vi "Excel___Write Channel Grouping.vi"(0 "Sheets Ref In":refnum<k7>, 5 "Starting Row":i32, 7 "Data 1":string[][](array[string]), 9 "Data 2":string[][](array[string]), 11 "Error In":errorcluster) -> (4 "Sheets Ref Out":refnum<k7>, 15 "Error Out":errorcluster)   [LabVIEW 2013]
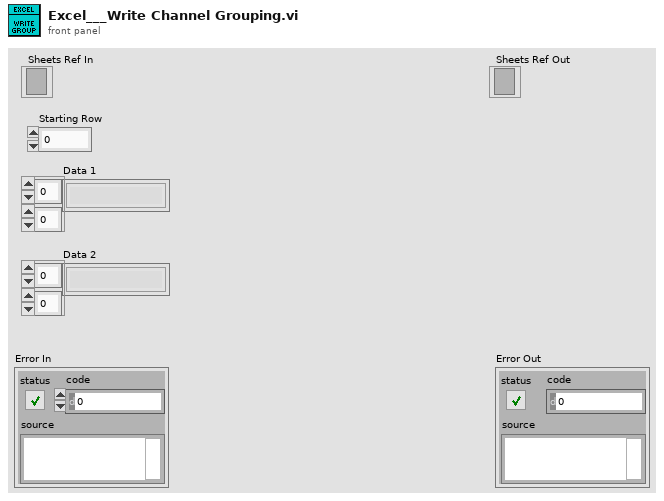
[diagram p1: front panel]
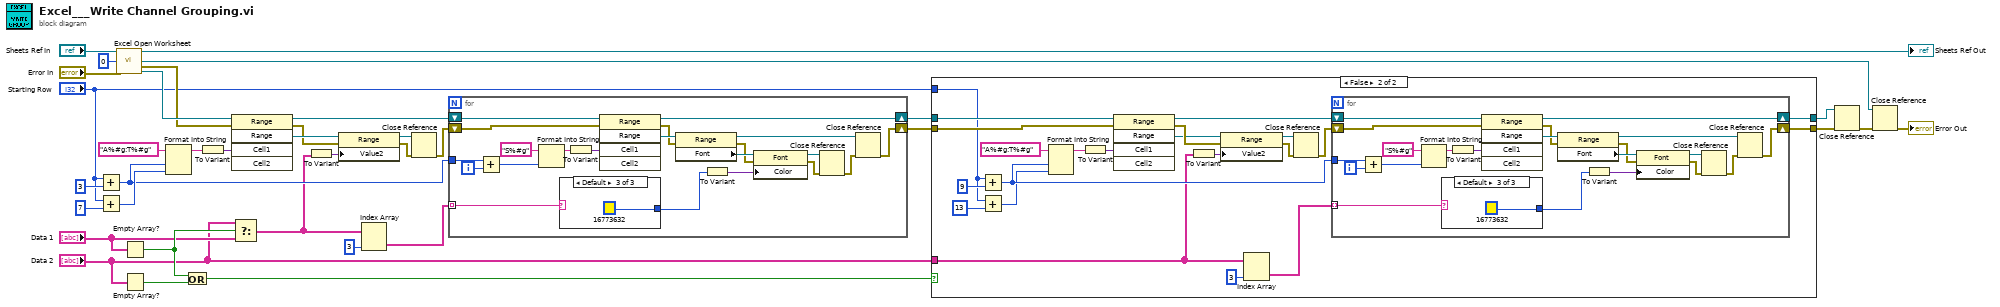
[diagram p0: block diagram]
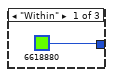
[diagram p3: hidden frame]
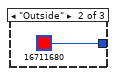
[diagram p4: hidden frame]
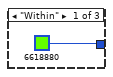
[diagram p5: hidden frame]
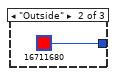
[diagram p6: hidden frame]
diagram:
  n1 = Add(x="Starting Row", y=3) -> (x+y=w13:i32)
  n2 = Add(x="Starting Row", y=7) -> (x+y=w19:i32)
  n3 = call "Excel Open Worksheet.vi"("Sheets Ref In"="Sheets Ref In", "Sheet#"=0, "Error In"="Error In") -> ("Sheets Ref Out"=→"Sheets Ref Out":refnum<k7>, "Worksheet Ref Out"=w27:refnum<k7>, "Error Out"=w23:errorcluster, "Cells Ref Out"=w24:refnum<k7>)  [unwired: 9 in]
  n4 = Empty Array?(array="Data 1") -> (empty?=w4:bool)
  n5 = Empty Array?(array="Data 2") -> (empty?=w6:bool)
  n6 = Format Into String(initial string="A%#g:T%#g", w13, w19) -> (resulting string=w35:string)  [unwired: 2 in, 1 out]
  n7 = Or(x=w4, y=w6) -> (x .or. y?=w5:bool)
  n8 = To Variant(anything=w35) -> (Variant=w34:variant)
  n9 = invoke class="Range" method="Range"(reference=w24, error in=w23, "Cell1"=w34) -> (reference out=w16:refnum<k7>, error out=w31:errorcluster, "Range"=w33:refnum<k7>)  [unwired: 2 in, 2 out]
  n10 = Select(t="Data 2", s=w4, f="Data 1") -> (s? t:f=w1:string[][])
  n11 = To Variant(anything=w1) -> (Variant=w32:variant)
  n12 = property class="Range"(reference=w33, error in=w31, "Value2"=w32) -> (reference out=w22:refnum<k7>, error out=w17:errorcluster)
  n13 = Index Array(array=w1, index (col)=3 ("disabled index (col)")) -> (element=w14:string[])  [unwired: 1 in]
  n14 = Close Reference(reference=w22, error in (no error)=w17) -> (error out=w15:errorcluster)
  n15 = for {
    tunnel: w14 -> [w46] mode=indexing
    shift-right: [w49] -> w12
    shift-left: w16 -> [w57]
    shift-right: [w37] -> w11
    shift-left: w15 -> [w56]
    tunnel: w13 -> [w53]
    i -> [w52]
    n16 = Add(x=w53, y=w52) -> (x+y=w51:i32)
    n17 = Format Into String(initial string="S%#g", w51) -> (resulting string=w55:string)  [unwired: 2 in, 1 out]
    n18 = case shown="Default" w46 {
      tunnel: [u32 6618880 u32 16711680 u32 16773632] -> w44
      frame "Within" {
      }
      frame "Outside" {
      }
      frame Default {
      }
    }
    n19 = To Variant(anything=w55) -> (Variant=w50:variant)
    n20 = invoke class="Range" method="Range"(reference=w57, error in=w56, "Cell1"=w50) -> (reference out=w49:refnum<k7>, error out=w43:errorcluster, "Range"=w48:refnum<k7>)  [unwired: 2 in, 2 out]
    n21 = property class="Range"(reference=w48, error in=w43) -> (reference out=w39:refnum<k7>, error out=w42:errorcluster, "Font"=w47:refnum<k7>)
    n22 = To Variant(anything=w44) -> (Variant=w45:variant)
    n23 = property class="Font"(reference=w47, error in=w42, "Color"=w45) -> (reference out=w40:refnum<k7>, error out=w41:errorcluster)
    n24 = Close Reference(reference=w40, error in (no error)=w41) -> (error out=w38:errorcluster)
    n25 = Close Reference(reference=w39, error in (no error)=w38) -> (error out=w37:errorcluster)
  }
  n26 = case shown="False" w5 {
    tunnel: [w62 w68] -> w10
    tunnel: w12 -> [w62 w67]
    tunnel: w11 -> [w61 w66]
    tunnel: [w61 w65] -> w8
    tunnel: "Data 2" -> [_ w64]
    tunnel: "Starting Row" -> [_ w63]
    frame True {
    }
    frame False {
      n27 = Add(x=w63, y=9) -> (x+y=w84:i32)
      n28 = Add(x=w63, y=13) -> (x+y=w78:i32)
      n29 = Format Into String(initial string="A%#g:T%#g", w84, w78) -> (resulting string=w70:string)  [unwired: 2 in, 1 out]
      n30 = To Variant(anything=w70) -> (Variant=w71:variant)
      n31 = invoke class="Range" method="Range"(reference=w67, error in=w66, "Cell1"=w71) -> (reference out=w81:refnum<k7>, error out=w74:errorcluster, "Range"=w72:refnum<k7>)  [unwired: 2 in, 2 out]
      n32 = To Variant(anything=w64) -> (Variant=w73:variant)
      n33 = property class="Range"(reference=w72, error in=w74, "Value2"=w73) -> (reference out=w75:refnum<k7>, error out=w80:errorcluster)
      n34 = Index Array(array=w64, index (col)=3 ("disabled index (col)")) -> (element=w83:string[])  [unwired: 1 in]
      n35 = Close Reference(reference=w75, error in (no error)=w80) -> (error out=w82:errorcluster)
      n36 = for {
        tunnel: w83 -> [w94] mode=indexing
        shift-right: [w97] -> w68
        shift-left: w81 -> [w105]
        shift-right: [w85] -> w65
        shift-left: w82 -> [w104]
        tunnel: w84 -> [w101]
        i -> [w100]
        n37 = Add(x=w101, y=w100) -> (x+y=w99:i32)
        n38 = Format Into String(initial string="S%#g", w99) -> (resulting string=w103:string)  [unwired: 2 in, 1 out]
        n39 = case shown="Default" w94 {
          tunnel: [u32 6618880 u32 16711680 u32 16773632] -> w92
          frame "Within" {
          }
          frame "Outside" {
          }
          frame Default {
          }
        }
        n40 = To Variant(anything=w103) -> (Variant=w98:variant)
        n41 = invoke class="Range" method="Range"(reference=w105, error in=w104, "Cell1"=w98) -> (reference out=w97:refnum<k7>, error out=w91:errorcluster, "Range"=w96:refnum<k7>)  [unwired: 2 in, 2 out]
        n42 = property class="Range"(reference=w96, error in=w91) -> (reference out=w87:refnum<k7>, error out=w90:errorcluster, "Font"=w95:refnum<k7>)
        n43 = To Variant(anything=w92) -> (Variant=w93:variant)
        n44 = property class="Font"(reference=w95, error in=w90, "Color"=w93) -> (reference out=w88:refnum<k7>, error out=w89:errorcluster)
        n45 = Close Reference(reference=w88, error in (no error)=w89) -> (error out=w86:errorcluster)
        n46 = Close Reference(reference=w87, error in (no error)=w86) -> (error out=w85:errorcluster)
      }
    }
  }
  n47 = Close Reference(reference=w10, error in (no error)=w8) -> (error out=w9:errorcluster)
  n48 = Close Reference(reference=w27, error in (no error)=w9) -> (error out=→"Error Out":errorcluster)
